vi "CopySelectedCells.vi"(6 "Clipboard":refnum<vi>, 8 "error in (no error)":errorcluster, 9 "Table CtlRef In":refnum<vi>) -> (0 "error out":errorcluster, 1 "Table CtlRef Out":refnum<vi>)   [LabVIEW 2013]
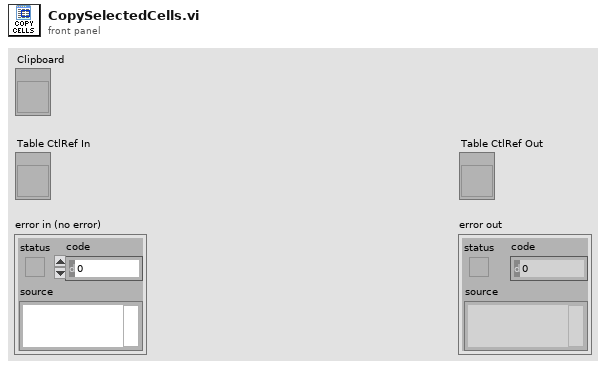
[diagram p1: front panel]
types:
  T1 = typedef "LVRowAndColumnTypeDef.ctl" = cluster{"Row":i32, "Column":i32}
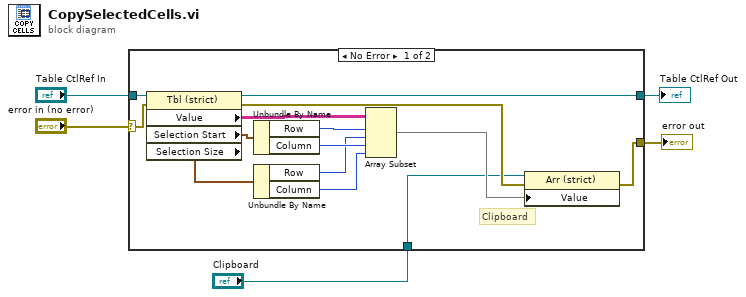
[diagram p0: block diagram]
diagram:
  n1 = case shown="No Error" "error in (no error)" {
    selector: "error in (no error)" -> [w6 w20]
    tunnel: "Table CtlRef In" -> [w10 w21]
    tunnel: "Clipboard" -> [w9 _]
    tunnel: [w8 w21] -> w3
    tunnel: [w7 w20] -> w2
    frame No Error {
      # "Clipboard"
      n2 = property class="Tbl (strict)"(reference=w10, error in=w6) -> (reference out=w8:refnum<vi>, error out=w11:errorcluster, "Value"=w18:string[][], "Selection Start"=w16:T1, "Selection Size"=w17:T1)
      n3 = Unbundle By Name(w16) -> ("Row"=w15:i32, "Column"=w14:i32)
      n4 = Unbundle By Name(w17) -> ("Row"=w13:i32, "Column"=w12:i32)
      n5 = Array Subset "Array Subset"(array=w18, index (row)=w15, length (row)=w13, index (col)=w14, length (col)=w12) -> (w19:string[][])
      n6 = property class="Arr (strict)"(reference=w9, error in=w11, "Value"=w19) -> (error out=w7:errorcluster)  [unwired: 1 out]
    }
    frame Error {
    }
  }
  "error out" <- w2
  "Table CtlRef Out" <- w3
